vi "Lvi Thermistor Channel Settings.vi"(0 "TaskRef":i32, 1 "C":dbl, 2 "DataFilter":u32, 5 "Channel":u32, 7 "A":dbl, 9 "B":dbl, 11 "error in (no error)":errorcluster, 12 "NumWireType":u32) -> (4 "TaskRef out":i32, 6 "function return":u32(ring), 15 "error out":errorcluster)   [LabVIEW 2022 SP3, in "DtLvLink.lvlib"]
doc: "Calls directly into the entry points of the DLL of the Data Acq SDK to set the configuration options for a thermistor measurement."
uses:
  DtLvLink.lvlib
  <userlib>/LV-Link3/DtLvLink_64.dll
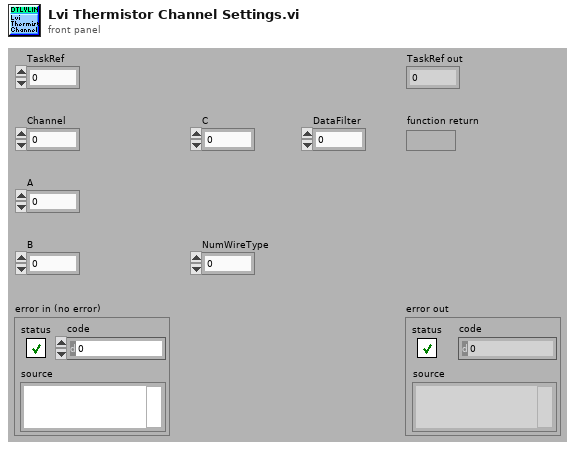
[diagram p1: front panel]
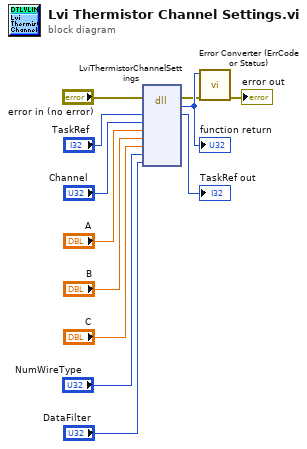
[diagram p0: block diagram]
diagram:
  n1 = dll-call lib="C:/Program Files/National Instruments/LabVIEW 2022/user.lib/LV-Link3/DtLvLink_64.*" fn="LviThermistorChannelSettings"(error in="error in (no error)", "TaskRef"="TaskRef", "Channel"="Channel", "A"="A", "B"="B", "C"="C", "NumWireType"="NumWireType", "DataFilter"="DataFilter") -> (error out=w2:errorcluster, w12:u32, "TaskRef"=→"TaskRef out":i32)  [unwired: 8 in, 1 out]
  "function return" <- w12
  n2 = call "Error Converter (ErrCode or Status).vi"("error in (no error)"=w2, "error code"=w12) -> ("error out"=→"error out":errorcluster)  [unwired: 9 in]
